vi "Save File to Project Directory.vi"(8 "错误输入":errorcluster, 10 "Sub Dir":string, 11 "Select VI":path) -> (0 "错误输出":errorcluster)   [LabVIEW 2011]
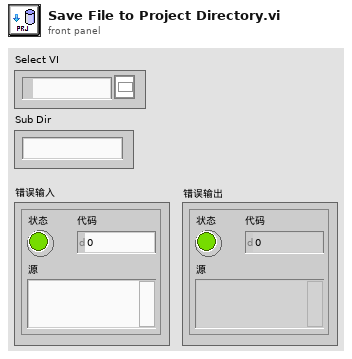
[diagram p1: front panel]
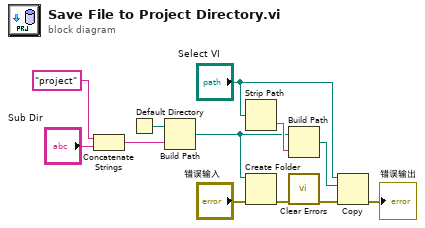
[diagram p0: block diagram]
diagram:
  n1 = Concatenate Strings("project" ("名称或相对路径"), "Sub Dir") -> (w3:string)
  n2 = Default Directory() -> (w12:path)
  n3 = Build Path(base path=w12, name or relative path=w3) -> (appended path=w1:path)
  n4 = Strip Path(path="Select VI") -> (name=w11:string)  [unwired: 1 out]
  n5 = Create Folder(path (use dialog)=w1, error in="错误输入") -> (error out=w7:errorcluster)  [unwired: 1 in, 2 out]
  n6 = Build Path(base path=w1, name or relative path=w11) -> (appended path=w8:path)
  n7 = call <vilib>:"Clear Errors.vi"("error in (no error)"=w7) -> ("error out"=w2:errorcluster)  [unwired: 6 in]
  n8 = Copy(8:w2, 10:w8, 11:"Select VI") -> (0:→"错误输出":errorcluster)  [unwired: 2 in, 2 out]
